vi "Wait for Key Release.vi"(8 "error in (no error)":errorcluster, 11 "Keyboard":refnum<k1>) -> (0 "error out":errorcluster, 3 "Keyboard out":refnum<k1>)   [LabVIEW 2020, in "MacroAssert.lvlib"]
doc: "Holds in a loop until all keys of <B>Keyboard</B> have been released (or an error occurs) before continuing."
uses:
  MacroAssert.lvlib
  <vilib>/Utility/inputDevices.llb/keyboardAcquire.vi
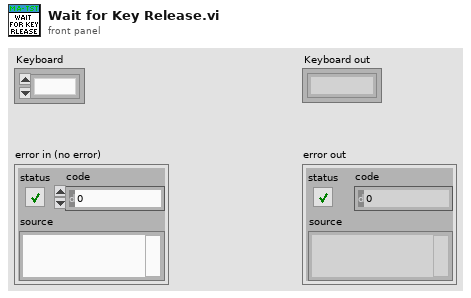
[diagram p1: front panel]
types:
  T1 = enum16{"0", "1", "2", "3", "4", "5", "6", "7", "8", "9", "A", "B", "C", "D", "E", "F", "G", "H", "I", "J", "K", "L", "M", "N", "O", "P", "Q", "R", "S", "T", "U", "V", "W", "X", "Y", "Z", "F1", "F2", "F3", "F4", "F5", "F6", "F7", "F8", "F9", "F10", "F11", "F12", "F13", "F14", "F15", "ADD", "BACK", "BACKSLASH", "CAPITAL", "COMMA", "DECIMAL", "DELETE", "DIVIDE", "DOWN", "END", "EQUALS", "ESCAPE", "GRAVE (`)", "HOME", "INSERT", "LBRACKET", "LCONTROL", "LEFT", "L ALT", "LSHIFT", "LWIN", "MINUS", "MULTIPLY", "NEXT", "NUMLOCK", "NUMPAD_0", "NUMPAD_1", "NUMPAD_2", "NUMPAD_3", "NUMPAD_4", "NUMPAD_5", "NUMPAD_6", "NUMPAD_7", "NUMPAD_8", "NUMPAD_9", "PAUSE", "PERIOD", "PRIOR (PG UP)", "RBRACKET", "RCONTROL", "RETURN", "RIGHT", "R ALT", "RSHIFT", "RWIN", "SCROLL", "SEMICOLON", "SLASH", "SPACE", "SUBTRACT", "TAB", "UP", "ENTER (num pad)", "' (quote)"}[]
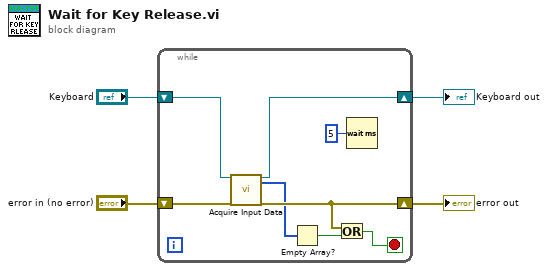
[diagram p0: block diagram]
diagram:
  n1 = while {
    shift-right: [w10] -> w2
    shift-left: "Keyboard" -> [w9]
    shift-right: [w11] -> w3
    shift-left: "error in (no error)" -> [w12]
    stop <- w7 stop-if-true
    n2 = call-poly <vilib>:"Acquire Input Data.vi"("device ID"=w9, "error in (no error)"=w12) -> ("device ID"=w10:refnum<k1>, "keys pressed"=w8:T1, "error out"=w11:errorcluster)  [unwired: 15 in]
    n3 = Empty Array?(array=w8) -> (empty?=w6:bool)
    n4 = Or(x=w11, y=w6) -> (x .or. y?=w7:bool)
    n5 = Wait (ms)(milliseconds to wait=u32 5) -> ()  [unwired: 1 out]
  }
  "error out" <- w3
  "Keyboard out" <- w2
